vi "Send and recieve IQ signals.vi"() -> ()   [LabVIEW 2019]
uses:
  SubVIs/mmWave HW Control/mmWave HW Control.lvlib
  <vilib>/Analysis/NI_AALPro.lvlib
  <instrlib>/niMmWave/ni3610 and ni3630/ni3610_and_ni3630_Driver_Lib.lvlib
  <vilib>/Analysis/2dsp.llb/1D Convolution (CDB).vi
  <vilib>/Analysis/4window.llb/windowTd.ctl
  SubVIs/Low-level/TypeDefs/Direction.ctl
  <vilib>/userdefined/High Color/nirio_resource_hc.ctl
  SubVIs/Low-level/TypeDefs/Resources.ctl
  SubVIs/Low-level/TypeDefs/Front End Configuration.ctl
  SubVIs/Low-level/TypeDefs/Channel Configuration.ctl
  SubVIs/Low-level/TypeDefs/Detected mmWave Adapters.ctl
  SubVIs/Low-level/TypeDefs/mmWave Adapter Information.ctl
  SubVIs/Low-level/TypeDefs/Hardware Configuration.ctl
  <instrlib>/niMmWave/ni3620/Config/v1/Host/Public/Typedefs/mmWave Port.ctl
  <instrlib>/niMmWave/ni3620/Config/v1/Host/niMmWave Config v1 Host.lvlib
  <instrlib>/niMmWave/ni3610 and ni3630/private/mm/Typedefs/PID.ctl
  <instrlib>/niMmWave/ni3610 and ni3630/controls/private/Board Hardware Revision.ctl
  <instrlib>/niMmWave/ni3610 and ni3630/controls/public/Board Information.ctl
  FPGA/SubVIs/Utility/FPGA driver trigger source.ctl
  FPGA/SubVIs/Utility/FPGA Utility.lvlib
  FPGA/SubVIs/Utility/FPGA driver trigger destination.ctl
  SubVIs/Low-level/TypeDefs/TX trigger config.ctl
panel:
  out "RX-TX delay":dbl format="%#.3ps"
  out "compensated max":i32
  out "max index":i32
  out "debug":u16
  out "debug.trig.count":u16
  out "time stamp out":timestamp
  out "State":string
  in  "indicators tab":T1(tab)=enum."Status"
  out "time domain":dbl[][](graph)
  in  "update graph":bool=TRUE
  in  "Scale":bool
  out "dt":dbl format="%#.3ps"
  out "frequency domain":cluster{"Ramp Pattern":dbl[], dbl[]}[](graph)
  in  "window":T2=8 items=["Rectangle"=0, "Hanning"=1, "Hamming"=2, "Blackman-Harris"=3, "Exact Blackman"=4, "Blackman"=5, "Flat Top"=6, "4 Term B-Harris "=7, "7 Term B-Harris"=8, "Low Sidelobe"=9, "Blackman Nuttall"=11, "Triangle"=30, "Bartlett-Hanning"=31, "Bohman"=32, "Parzen"=33, "Welch"=34, "Kaiser"=60, "Dolph-Chebyshev"=61, "Gaussian"=62]
  out "bandwidth (Hz)":dbl[](array[numeric]) format="%#_6p"
  out "Tx information":T3={"product code"=30638, "hardware revision"=enum."B", "serial number"="MTX1008\u0000"} {"product code" items=["PXIe-3610 I/Q Generator"=30638, "PXIe-3630 I/Q Digitizer"=30639]}
  out "Rx information 2":T3={"product code"=30638, "hardware revision"=enum."B", "serial number"="MTX1008\u0000"} {"product code" items=["PXIe-3610 I/Q Generator"=30638, "PXIe-3630 I/Q Digitizer"=30639]}
  out "coerced device configuration [channel]":T6[](array[typedef])=[{"port select"=enum."IF Port", "Rx hardware configuration"={"gain (dB)"=24.131681691521095, "frequency (Hz)"=71000000000.0, "mmWave adapter"="mmWave0/0", "adapter active port"="RX1"}, "Tx hardware configuration"={"gain (dB)"=0.5400391534496903, "frequency (Hz)"=71000000000.0, "mmWave adapter"="mmWave1/0", "adapter active port"="TX1"}}] {"Tx hardware configuration"."frequency (Hz)" format="%#_6p"; "Rx hardware configuration"."frequency (Hz)" format="%#_6p"}
  out "detected mmWave adapters [channel]":T9[](array[typedef])=[{"3620 resource name"="IF_mod_demod", "detected mmWave adapters"=[{"scope"="mmWave0/0", "mmWave adapter type"="NI 3657 71-76 GHz Rx Downconverter", "serial number"=12322}, {"scope"="mmWave1/0", "mmWave adapter type"="NI 3647 71-76 GHz Tx Upconverter", "serial number"=12292}]}] {"detected mmWave adapters"."serial number" format="%.0x"}
  out "error out":errorcluster
  in  "Trig share":T12(tab)
  in  "Sync module (export)":tag="PXI2Slot2"
  in  "Export PXI trigger":string(combo)="PXI_Trig0"
  in  "Sync module export terminal":string(combo)="PFI0"
  in  "Sync module import terminal":string(combo)="PFI0"
  in  "Import PXI trigger":string(combo)="PXI_Trig0"
  in  "Sync module (import)":tag="PXI2Slot2"
  in  "stop":bool
  in  "controls tab":enum32{"Setup", "Hardware", "Application"}(tab)=enum."Hardware"
  in  "option string":string="sample_rate=3.072G"
  in  "hardware resources [channel]":T13[](array[typedef])=[{"7902R (Tx)"="Tx_FPGA", "3610 (Tx)"="Tx_DAC", "3620 (IF)"="IF_mod_demod", "3630 (RX)"="Rx_ADC", "7902R (Rx)"="Rx_FPGA"}]
  in  "hardware setup":T14
  in  "update hardware settings":bool
  in  "device configuration [channel]":T6[](array[typedef])=[{"port select"=enum."IF Port", "Rx hardware configuration"={"gain (dB)"=0.0, "frequency (Hz)"=76000000000.0, "mmWave adapter"="mmWave0/0", "adapter active port"="RX1"}, "Tx hardware configuration"={"gain (dB)"=-10.0, "frequency (Hz)"=76000000000.0, "mmWave adapter"="mmWave1/0", "adapter active port"="TX1"}}] {"Tx hardware configuration"."frequency (Hz)" format="%#_6p"; "Rx hardware configuration"."frequency (Hz)" format="%#_6p"}
  in  "TX trigger options":T16
  in  "RX trigger options":T16={"delay"=158.0, "trig source"=enum."Use Tclk", "PXI src"=0, "export"=enum."None", "PXI dest"=1}
  in  "acquisition samples":u32=16000
  in  "digital gain (dB)":dbl format="%#_13g"
  in  "update app settings":bool
  in  "IQ signal":cdb[](array[numeric])=[1.0+0.0i]
  in  "IQ rate":dbl=50000000.0 format="%#_6p"
  in  "signal length":i32=1600
  in  "trigger pulse":bool
  in  "gen.burst/cont":bool=TRUE
  in  "Timeout (ms)":i32=5000
  # "Instructions:\n(1) Select device resources (Setup tab)\n(2) Select hardware setup (Setup tab)\n(3) Set device configuration\n         See datasheet for recommended gain settings\n          Warning: Incompatible gain settings may damage hardware.  \n                         Refer to datasheet for recommended gain settings.\n(4) Run this example\n\nNote: The Receiver and Transmitter must be connected (loopback) and the hardware configuration must be set\nto transceiver in order for channel equalization to occur.  When looping back at mmWave, be sure to \nconsult the datasheet to ensure sufficient path loss."
  # "no trigger sharing through timing module"
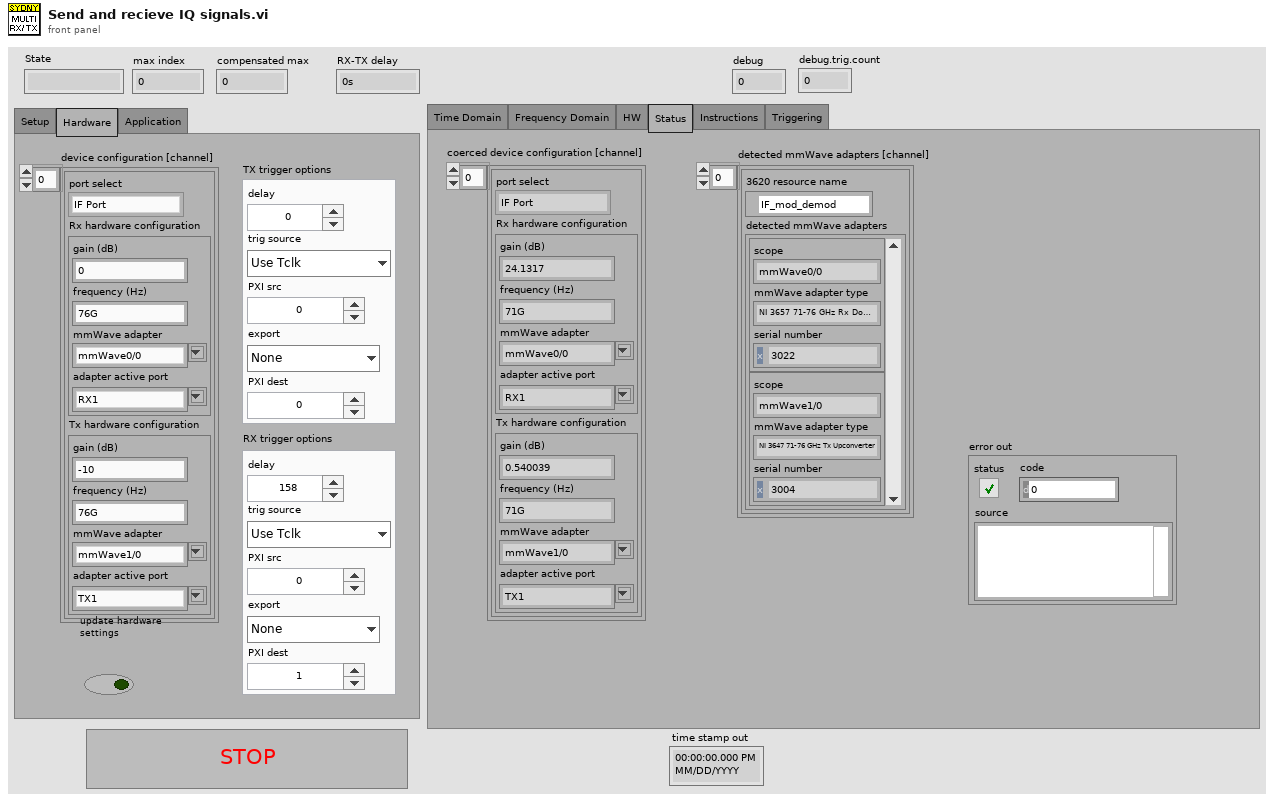
[diagram p1: front panel]
types:
  T1 = enum32{"Time Domain", "Frequency Domain", "HW", "Status", "Instructions", "Triggering"}
  T2 = typedef "NI_AALPro.lvlib/windowTd.ctl" = u32
  T3 = typedef "Board Information.ctl" = cluster{"product code":T4, "hardware revision":T5, "serial number":string}
  T4 = typedef "ni3610_and_ni3630_Driver_Lib.lvlib/PID.ctl" = u16
  T5 = typedef "Board Hardware Revision.ctl" = enum16{"Unknown", "A", "B", "C", "D", "E", "F", "G", "H"}
  T6 = typedef "Front End Configuration.ctl" = cluster{"port select":enum16{"IF Port", "Loopback", "Sync Port"}, "Rx hardware configuration":T7, "Tx hardware configuration":T7}
  T7 = typedef "Channel Configuration.ctl" = cluster{"gain (dB)":dbl, "frequency (Hz)":dbl, "mmWave adapter":string, "adapter active port":T8}
  T8 = typedef "niMmWave Config v1 Host.lvlib/mmWave Port.ctl" = string
  T9 = typedef "Detected mmWave Adapters.ctl" = cluster{"3620 resource name":T10, "detected mmWave adapters":T11[]}
  T10 = typedef "nirio_resource_hc.ctl" = tag
  T11 = typedef "mmWave Adapter Information.ctl" = cluster{"scope":string, "mmWave adapter type":string, "serial number":u64}
  T12 = enum32{"No trig share", "Export trig", "Import trig"}
  T13 = typedef "Resources.ctl" = cluster{"7902R (Tx)":T10, "3610 (Tx)":refnum<visa-resource-name>, "3620 (IF)":T10, "3630 (RX)":refnum<visa-resource-name>, "7902R (Rx)":T10}
  T14 = typedef "Hardware Configuration.ctl" = cluster{"direction":T15, "baseband only":bool}
  T15 = typedef "Direction.ctl" = enum16{"Transceiver", "Receiver", "Transmitter"}
  T16 = typedef "TX trigger config.ctl" = cluster{"delay":dbl, "trig source":T17, "PXI src":i32, "export":T18, "PXI dest":i32}
  T17 = typedef "FPGA Utility.lvlib/FPGA driver trigger source.ctl" = enum16{"Use Tclk", "PXI_Trig", "Aurora RX trig"}
  T18 = typedef "FPGA Utility.lvlib/FPGA driver trigger destination.ctl" = enum16{"None", "Source trig", "Synced trig", "Delayed sync"}
  T19 = typedef "Session.ctl" = cluster{"3620 session":refnum<queue>, "tx baseband session":T20, "rx baseband session":T28, "tx gain (dB)":dbl, "rx gain (dB)":dbl, "hardware configuration":T14, "gain ranging":T29[], "pxi trigger bus information":T30}
  T20 = typedef "Tx Baseband Session.ctl" = cluster{"3610 session":T21, "7902 reference":T27}
  T21 = typedef "ni3610_and_ni3630_Driver_Lib.lvlib/Main Settings.ctl" = cluster{"VISA resource name":refnum<visa-resource-name>, "Address Space":T22, "window_offset":u32, "register_addresses":T23, "required_MM_fpga_version":cluster{"signature":u32, "hardware":u32, "current revision":u32, "oldest revision":u32}, "CPLD Oldest Compat Version ":cluster{"hardware":u32, "CPLD firmware":u32}, "MM_FPGA_image_location":string, "is_init":bool, "card_type":T24, "DacLmkConfigFileName":string, "AdcLmkConfigFileName":string, "AdcConfigFileName":string, "DacConfigFileName_RevA":string, "DacConfigFileName_RevB":string, "Mulde hardware revision":u8, "bypass DAC PLL\n":bool, "IQ Card Revision":T25, "board capability":T26}
  T22 = typedef "VISA Register Access Address Space.ctl" = u16
  T23 = typedef "ni3610_and_ni3630_Driver_Lib.lvlib/Register Adresses.ctl" = cluster{"MM based Registers":cluster{"Revision":u32, "OldestCompatRev":u32, "signature":u32, "scratch":u32, "LedControl":u32, "BoardHwRev":u32, "BoardControl":u32, "ThermalStatus":u32, "BasebandStatus":u32, "BasebandControl":u32, "BasebandAuxSetup":u32, "BasebandAuxStatus":u32, "LmkSyncOutSetup":u32, " AdcSyncOutSetup":u32, " InjSyncOutSetup":u32, " PxiTrig0OutSetup":u32, " PxiTrig1OutSetup":u32, " PxiTrig2OutSetup":u32, " PxiTrig3OutSetup":u32, " PxiTrig4OutSetup":u32, " PxiTrig5OutSetup":u32, " PxiTrig6OutSetup":u32, " PxiTrig7OutSetup":u32}, "CPLD based Registers":cluster{"SlaveSignature":u32, "SlaveRevision":u32, "SlaveOldestCompatRev":u32, "SlaveScratch":u32, "SlaveSetup":u32, "SlaveStatus":u32, "IDacReg_offset":u32, "LMKRegGrp0_offset":u32, "QDacReg_offset":u32, "BrdTempSensorVal":u32, "TempSensorPowerDown":u32, "GPIOReg_offset":u32, "IAdcReg_offset":u32, "QAdcReg_offset":u32, "LMKRegGrp1_offset":u32, "QadcTempSensorVal":u32, "IadcTempSensorVal":u32, "RevisionReg":u32, "VcxoReg":u32, "CpldStatusReg":u32, "PowerReg":u32, "VBiasEnReg":u32, "ExtRefOeReg":u32, "QdacCtrlReg":u32, "QdacStatusReg":u32, "IdacCtrlReg":u32, "IdacStatusReg":u32, "QdacJtagIn":u32, "QdacJtagOut":u32, "IdacJtagIn":u32, "IdacJtagOut":u32, "IqDcSetupReg":u32, "QadcStatusReg":u32, "IadcStatusReg":u32, "BrdSetupReg":u32, "IqDcRevisionReg":u32, "PllStatusReg":u32, "EndpointScratchReg":u32, "AdcSyncCfgReg":u32, "IqCardOpampReg":u32}, "CPLD Register Offset":u32, "MM  Register Offset":u32, " PxiTrig0OutSetup":u32}
  T24 = typedef "ni3610_and_ni3630_Driver_Lib.lvlib/Base Card Type.ctl" = enum16{"unspecified", "ADC", "DAC"}
  T25 = typedef "ni3610_and_ni3630_Driver_Lib.lvlib/IQ Card Revision.ctl" = enum16{"RevA", "RevB", "RevC", "RevD"}
  T26 = typedef "ni3610_and_ni3630_Driver_Lib.lvlib/Board Capability.ctl" = cluster{"baseband sync":enum16{"no baseband sync", "baseband sync"}}
  T27 = typedef "Blank FPGA Reference.ctl" = refnum<k20>
  T28 = typedef "Rx Baseband Session.ctl" = cluster{"3630 session":T21, "7902 reference":T27}
  T29 = typedef "Gain Ranging.ctl" = cluster{"gain ranging active scope":string, "gain ranging stream session":refnum<k20>}
  T30 = typedef "PXI Trigger Bus Info.ctl" = cluster{"chassis resource name":refnum<visa-resource-name>, "7902R (TX)":i16, "3610 (TX)":i16, "3620 (IF)":i16, "3630 (RX)":i16, "7902R (RX)":i16}
  T31 = cluster{"Sync module import terminal":string, "Import PXI trigger":string}
  T32 = cluster{"frequency offset (Hz)":dbl[], "response":cdb[]}[]
  T33 = cluster{"frequency offset (Hz)":dbl[], "response":cdb[]}
  T34 = typedef "Constants.ctl" = cluster{"data clock rate (Hz)":dbl, "sample rate (Hz)":dbl, "sample rate selector string":string, "default tx bitfile path":path, "default rx bitfile path":path, "default proc bitfile path":path}
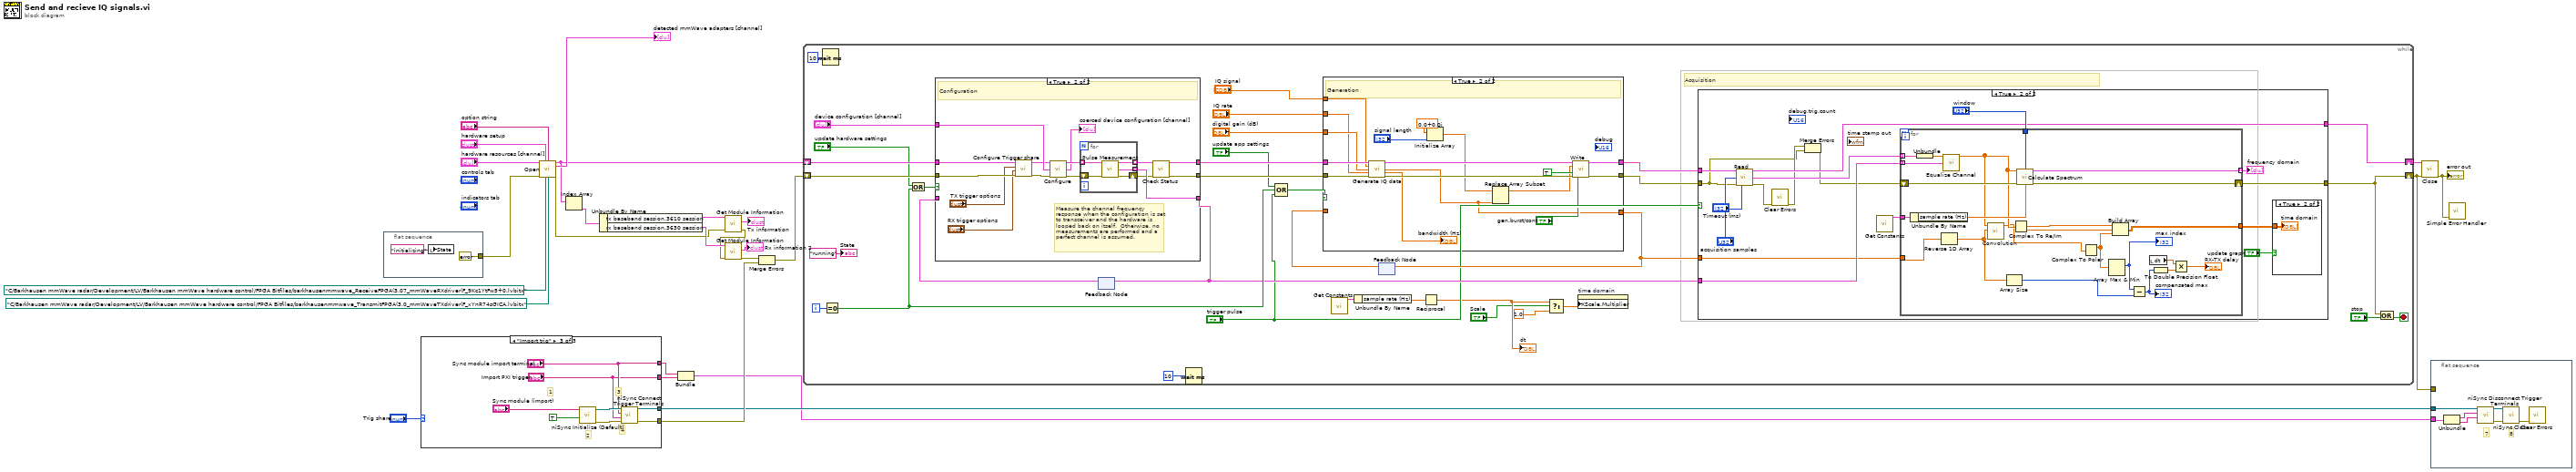
[diagram p0: block diagram]
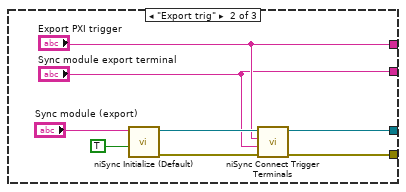
[diagram p3: hidden frame]
diagram:
  n1 = flat-sequence {
    tunnel: [errorcluster {"status"=FALSE, "code"=0, "source"=""} ("error constant")] -> w20
    frame #0 {
      n2 = local write "State"("initializing" ("State")) -> ()
    }
  }
  n3 = case shown="\"Import trig\"" "Trig share" {
    tunnel: [_ w34 w39] -> w4
    tunnel: [_ "Export PXI trigger" "Sync module import terminal"] -> w2
    tunnel: [_ "Sync module export terminal" "Import PXI trigger"] -> w3
    tunnel: [_ w29 w40] -> w6
    frame "No trig share", Default {
    }
    frame "Export trig" {
      n4 = call <instrlib>:"niSync Initialize (Default).vi"("reset device (F)"=TRUE ("reset device (False)"), "resource name"="Sync module (export)") -> ("error out"=w30:errorcluster, "instrument handle out"=w36:refnum<k15>)  [unwired: 8 in]
      n5 = call <instrlib>:"niSync Connect Trigger Terminals.vi"("error in (no error)"=w30, "destination terminal"="Sync module export terminal", "source terminal"="Export PXI trigger", "instrument handle"=w36) -> ("error out"=w29:errorcluster, "instrument handle out"=w34:refnum<k15>)  [unwired: 6 in]
    }
    frame "Import trig" {
      # "4"
      # "3"
      # "2"
      # "1"
      n6 = call <instrlib>:"niSync Initialize (Default).vi"("reset device (F)"=TRUE ("reset device (False)"), "resource name"="Sync module (import)") -> ("error out"=w44:errorcluster, "instrument handle out"=w42:refnum<k15>)  [unwired: 8 in]
      n7 = call <instrlib>:"niSync Connect Trigger Terminals.vi"("error in (no error)"=w44, "destination terminal"="Import PXI trigger", "source terminal"="Sync module import terminal", "instrument handle"=w42) -> ("error out"=w40:errorcluster, "instrument handle out"=w39:refnum<k15>)  [unwired: 6 in]
    }
  }
  n8 = call "Open.vi"("resources"="hardware resources [channel]", "hardware configuration"="hardware setup", "option string"="option string", "error in"=w20, "rx bitfile path"=path "C:/Barkhausen mmWave radar/Development/LV/Barkhausen mmWave hardware control/FPGA Bitfiles/barkhausenmmwave_ReceiveFPGA(3.07_mmWaveRXdriver(F_9Kc1YtFw5+0.lvbitx", "tx bitfile path"=path "C:/Barkhausen mmWave radar/Development/LV/Barkhausen mmWave hardware control/FPGA Bitfiles/barkhausenmmwave_TransmitFPGA(3.0_mmWaveTXdriver(F_xYnR74sGICA.lvbitx" ("rx bitfile path")) -> ("session out"=w12:T19[], "detected mmWave adapters"=→"detected mmWave adapters [channel]":T9[], "error out"=w11:errorcluster)  [unwired: 7 in]
  n9 = Index Array(array=w12) -> (element=w19:T19)  [unwired: 1 in]
  n10 = Unbundle By Name(w19) -> ("tx baseband session.3610 session"=w18:T21, "rx baseband session.3630 session"=w17:T21)
  n11 = Bundle("Sync module import terminal"=w2, "Import PXI trigger"=w3) -> (w1:T31)  [unwired: 1 in]
  n12 = call <instrlib>:"Get Module Information.vi"("error in (no error)"=w11, "Board Settings in"=w18) -> ("error out"=w10:errorcluster, "board information"=→"Tx information":T3)  [unwired: 7 in, 1 out]
  n13 = call <instrlib>:"Get Module Information.vi"("error in (no error)"=w10, "Board Settings in"=w17) -> ("error out"=w9:errorcluster, "board information"=→"Rx information 2":T3)  [unwired: 7 in, 1 out]
  n14 = Merge Errors(w9, w6) -> (w7:errorcluster)
  n15 = while {
    shift-right: [w59] -> w5
    shift-left: w7 -> [w66]
    shift-right: [w58] -> w26
    shift-left: w12 -> [w67]
    i -> [w74]
    stop <- w78 stop-if-true
    # "Acquisition"
    n16 = Wait (ms)(milliseconds to wait=u32 10) -> ()  [unwired: 1 out]
    n17 = Equal To 0?(x=w74) -> (x = 0?=w60:bool)
    n18 = Compound Arithmetic op=OR("update hardware settings", w60) -> (w68:bool)
    n19 = feedback #1() -> (w73:T32)  [unwired: 1 in]
    n20 = case shown="True" w68 {
      tunnel: w66 -> [w144 w149]
      tunnel: w67 -> [w143 w150]
      tunnel: [w144 w157] -> w70
      tunnel: "device configuration [channel]" -> [_ w152]
      tunnel: [w143 w156] -> w71
      tunnel: [w142 w159] -> w57
      tunnel: w73 -> [w142 _]
      frame False {
      }
      frame True {
        # "Measure the channel frequency\nresponse when the configuration is set\nto transceiver and the hardware is \nlooped back on itself.  Otherwise, no\nmeasurements are performed and a\nperfect channel is assumed."
        # "Configuration"
        n21 = call "Configure Trigger share.vi"("error in"=w149, "RX trigger options"="RX trigger options", "TX trigger options"="TX trigger options", "session in"=w150) -> ("error out"=w148:errorcluster, "session out"=w147:T19[])  [unwired: 4 in, 2 out]
        n22 = call "Configure.vi"("session in"=w147, "device configuration [channel]"=w152, "error in"=w148) -> ("session out"=w154:T19[], "coerced device configuration [channel]"=→"coerced device configuration [channel]":T6[], "error out"=w153:errorcluster)  [unwired: 10 in]
        n23 = for {
          shift-right: [w163] -> w158
          shift-left: w153 -> [w160]
          tunnel: w154 -> [w161] mode=indexing
          tunnel: [w164] -> w155 mode=indexing
          tunnel: [w162] -> w159 mode=indexing
          n24 = call "Pulse Measurement.vi"("session"=w161, "error in"=w160) -> ("session out"=w164:T19, "channel"=w162:T33, "error out"=w163:errorcluster)  [unwired: 11 in]
        }
        n25 = call "Check Status.vi"("session in"=w155, "error in"=w158) -> ("session out"=w156:T19[], "error out"=w157:errorcluster)  [unwired: 9 in, 3 out]
      }
    }
    n26 = feedback-in #1(w57) -> ()
    n27 = Wait (ms)(milliseconds to wait=u32 10) -> ()  [unwired: 1 out]
    n28 = Compound Arithmetic op=OR("update app settings", w60, "trigger pulse") -> (w63:bool)
    n29 = call "Get Constants.vi"() -> ("constants"=w49:T34)  [unwired: 15 in]
    n30 = Unbundle By Name(w49) -> ("sample rate (Hz)"=w48:dbl)
    n31 = feedback #2() -> (w54:cdb[])  [unwired: 1 in]
    n32 = case shown="True" w63 {
      tunnel: [w123 w141] -> w75
      tunnel: w70 -> [w123 w139]
      tunnel: [w124 w140] -> w72
      tunnel: w71 -> [w124 w138]
      tunnel: "digital gain (dB)" -> [_ w134]
      tunnel: "IQ signal" -> [_ w133]
      tunnel: "IQ rate" -> [_ w132]
      tunnel: w54 -> [w122 _]
      tunnel: [w122 w126] -> w53
      frame False {
      }
      frame True {
        # "Generation"
        n33 = call "Generate IQ data.vi"("session in"=w138, "IQ signal"=w133, "digital gain (dB)"=w134, "IQ rate"=w132, "error in"=w139) -> ("session out"=w136:T19[], "IQ"=w126:cdb[], "bandwidth (Hz)"=→"bandwidth (Hz)":dbl[], "error out"=w137:errorcluster)  [unwired: 6 in, 1 out]
        n34 = Initialize Array(cdb 0.0+0.0i ("element"), "signal length") -> (w128:cdb[])
        n35 = Replace Array Subset(array=w128, new element=w126) -> (w125:cdb[])  [unwired: 1 in]
        n36 = call "Write.vi"("session in"=w136, "data"=w125, "zero pad"=TRUE, "error in"=w137, 12:"gen.burst/cont") -> ("session out"=w140:T19[], "error out"=w141:errorcluster)  [unwired: 7 in, 2 out]
      }
    }
    n37 = feedback-in #2(w53) -> ()
    n38 = Reciprocal(x=w48) -> (1/x=w47:dbl)
    "dt" <- w47
    n39 = Select(t=w47, s="Scale", f=1.0 ("X Scale.Offset and Multiplier:Multiplier")) -> (s? t:f=w46:dbl)
    n40 = property on="time domain" class="WFGraph (strict)"("XScale.Multiplier"=w46) -> ()  [unwired: 2 in, 2 out]
    n41 = case shown="True" "trigger pulse" {
      tunnel: w75 -> [w79 w82]
      tunnel: w72 -> [w80 w97]
      tunnel: [w79 w92] -> w59
      tunnel: [w80 w91] -> w58
      tunnel: w57 -> [_ w89]
      tunnel: w53 -> [_ w86]
      frame False {
      }
      frame True {
        n42 = call "Read.vi"("session in"=w97, "number of samples"="acquisition samples", "error in"=w82, "Timeout (ms)"="Timeout (ms)") -> ("session out"=w91:T19[], "data [channel]"=w90:cluster{"data":cdb[]}[], "error out"=w85:errorcluster)  [unwired: 9 in]
        n43 = call <vilib>:"Clear Errors.vi"("error in (no error)"=w85) -> ("error out"=w83:errorcluster)  [unwired: 5 in, 1 out]
        n44 = Merge Errors(w83, w82) -> (w84:errorcluster)
        n45 = call "Get Constants.vi"() -> ("constants"=w88:T34)  [unwired: 15 in]
        n46 = for {
          tunnel: [w121] -> w94
          tunnel: [w120] -> w95 mode=indexing
          tunnel: "window" -> [w119]
          shift-right: [w118] -> w92
          shift-left: w84 -> [w110]
          tunnel: w90 -> [w116] mode=indexing
          tunnel: w89 -> [w115] mode=indexing
          tunnel: w88 -> [w113]
          tunnel: w86 -> [w109]
          n47 = Unbundle By Name(w113) -> ("sample rate (Hz)"=w114:dbl)
          n48 = Unbundle(w116) -> ("data"=w117:cdb[])
          n49 = Reverse 1D Array(array=w109) -> (reversed array=w105:cdb[])
          n50 = call "Equalize Channel.vi"("input data"=w117, "channel"=w115) -> ("output data"=w108:cdb[])  [unwired: 12 in, 1 out]
          n51 = call-poly <vilib>:"Convolution.vi"("Y"=w105, "X"=w108) -> ("X * Y"=w107:cdb[])  [unwired: 8 in, 1 out]
          n52 = Array Size(array=w105) -> (size(s)=w103:i32)
          n53 = Complex To Re/Im(x + iy=w108) -> (x=w112:dbl[], y=w111:dbl[])
          n54 = call "Calculate Spectrum.vi"("input data"=w108, "window"=w119, "error in"=w110, "IQ rate"=w114) -> ("spectrum output"=w120:cluster{"Ramp Pattern":dbl[], dbl[]}, "error out"=w118:errorcluster)  [unwired: 10 in]
          n55 = Complex To Polar(r * e^(i*theta)=w107) -> (r=w106:dbl[])  [unwired: 1 out]
          n56 = Array Max & Min(array=w106) -> (max index (indices)=w104:i32)  [unwired: 3 out]
          "max index" <- w104
          n57 = Build Array(w112, w111, w106) -> (w121:dbl[][])
          n58 = Subtract(x=w104, y=w103) -> (x-y=w102:i32)
          "compensated max" <- w102
          n59 = local read "dt"() -> (w100:dbl)
          n60 = To Double Precision Float(number=w102) -> (double precision float=w101:dbl)
          n61 = Multiply(x=w100, y=w101) -> (x*y=→"RX-TX delay":dbl)
        }
        "frequency domain" <- w95
        n62 = case shown="True" "update graph" {
          tunnel: w94 -> [_ w98]
          frame False {
          }
          frame True {
            "time domain" <- w98
          }
        }
      }
    }
    n63 = Compound Arithmetic op=OR(w59, "stop") -> (w78:bool)
    "State" <- "running" ("State")
  }
  n64 = call "Close.vi"("session"=w26, "error in"=w5) -> ("error out"=w21:errorcluster)  [unwired: 13 in]
  "error out" <- w21
  n65 = flat-sequence {
    tunnel: w5 -> [_]
    tunnel: w4 -> [w168]
    tunnel: w1 -> [w167]
    frame #0 {
      # "8"
      # "7"
      n66 = Unbundle(w167) -> ("Sync module import terminal"=w166:string, "Import PXI trigger"=w165:string)
      n67 = call <instrlib>:"niSync Disconnect Trigger Terminals.vi"("destination terminal"=w165, "source terminal"=w166, "instrument handle"=w168) -> ("error out"=w171:errorcluster, "instrument handle out"=w170:refnum<k15>)  [unwired: 7 in]
      n68 = call <instrlib>:"niSync Close.vi"("error in (no error)"=w171, "instrument handle"=w170) -> ("error out"=w169:errorcluster)  [unwired: 9 in]
      n69 = call <vilib>:"Clear Errors.vi"("error in (no error)"=w169) -> ()  [unwired: 5 in, 2 out]
    }
  }
  n70 = call <vilib>:"Simple Error Handler.vi"("error in (no error)"=w21) -> ()  [unwired: 4 in, 5 out]
